vi "Test Remove Test from Suite.vi"(8 "error in (no error)":errorcluster, 11 "LUnit Test Suite Tests in":refnum<class "LUnit Test Suite Tests.lvclass">) -> (0 "error out":errorcluster, 3 "LUnit Test Suite Tests out":refnum<class "LUnit Test Suite Tests.lvclass">)   [LabVIEW 2020, in "LUnit Test Suite Tests.lvclass"]
uses:
  LUnit Test Suite Tests.lvclass
  C:/Program Files (x86)/National Instruments/LabVIEW 2020/vi.lib/Astemes/LUnit/Test Case.lvclass
  Test Doubles/Test Case Test Double/Methods.ctl
  <vilib>/Astemes/LUnit/Test Case.lvclass/Test Case.ctl
  <vilib>/Astemes/LUnit/Append Fail Result.vi
  <vilib>/Astemes/LUnit/Append Pass Result.vi
  source/API/LUnit Test Case/LUnit Test Case.lvclass
  C:/git/astemes-lunit/source/Core/Runnable/Runnable.lvclass
  LUnit Test Suite Tests.lvclass/LUnit Test Suite Tests.ctl
  Test Doubles/Test Case Test Double/Test Case Test Double.lvclass
  source/API/LUnit Test Suite/LUnit Test Suite.lvclass
  <vilib>/Astemes/LUnit/Test Case.lvclass
panel:
  out "List of Runnables":string[](array[string])
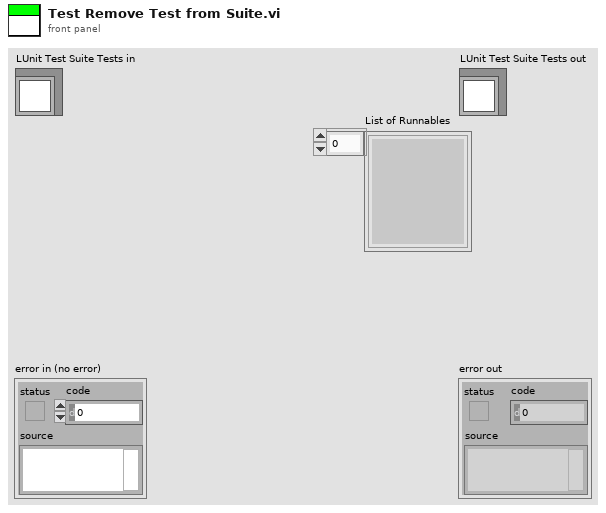
[diagram p1: front panel]
types:
  T1 = typedef "Test Case Test Double.lvclass/Methods.ctl" = enum16{"Test Failing Test.vi", "Test Passing Test.vi", "Test Error Test.vi", "Test Skip Test.vi", "Test Passing Pass If Test.vi", "Test Failing Pass If Test.vi", "Test Failing Fail If Test.vi", "Test Passing Fail If Test.vi", "Test Passing Pass If Error Test.vi", "Test Failing Pass If Error Test.vi", "Test Passing Fail If Error Test.vi", "Test Failing Fail If Error Test.vi", "Test Passing Pass If Equal Test.vi", "Test Failing Pass If Equal Test.vi", "Test Failing Fail If Equal Test.vi", "Test Passing Fail If Equal Test.vi", "Freezing Test.vi"}
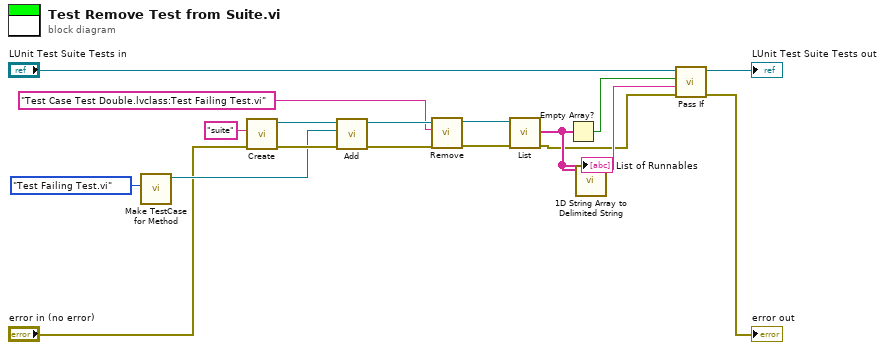
[diagram p0: block diagram]
diagram:
  n1 = call "Make TestCase for Method.vi"("Test Method"=Methods."Test Failing Test.vi") -> ("LUnit Test Case V2 out"=w14:refnum<class "LUnit Test Case.lvclass">)  [unwired: 9 in, 1 out]
  n2 = call "Create.vi"("error in (no error)"="error in (no error)", "Suite Name"="suite") -> ("error out"=w15:errorcluster, "LUnit Test Suite Out"=w16:refnum<class "LUnit Test Suite.lvclass">)  [unwired: 8 in]
  n3 = call "Add.vi"("error in (no error)"=w15, "Runnable"=w14, "LUnit Test Suite In"=w16) -> ("error out"=w11:errorcluster, "LUnit Test Suite Out"=w13:refnum<class "LUnit Test Suite.lvclass">)  [unwired: 7 in]
  n4 = call "Remove.vi"("error in (no error)"=w11, "Test to Remove"="Test Case Test Double.lvclass:Test Failing Test.vi" ("Name"), "LUnit Test Suite In"=w13) -> ("error out"=w9:errorcluster, "LUnit Test Suite Out"=w10:refnum<class "LUnit Test Suite.lvclass">)  [unwired: 7 in]
  n5 = call "List.vi"("error in (no error)"=w9, "LUnit Test Suite In"=w10) -> ("error out"=w2:errorcluster, "List of Runnables"=w4:string[])  [unwired: 8 in]
  "List of Runnables" <- w4
  n6 = Empty Array?(array=w4) -> (empty?=w5:bool)
  n7 = call <vilib>:"1D String Array to Delimited String.vi"("string array"=w4) -> ("delimited string"=w3:string)  [unwired: 10 in]
  n8 = call <vilib>:"Pass If.vi"("error in (no error)"=w2, "Message"=w3, "Pass?"=w5, "LUnit Test Case In"="LUnit Test Suite Tests in") -> ("error out"=→"error out":errorcluster, "LUnit Test Case Out"=→"LUnit Test Suite Tests out":refnum<class "LUnit Test Suite Tests.lvclass">)  [unwired: 6 in]
